vi "DDS_Clock.vi"() -> ()   [LabVIEW 2016] (continued)
CH0"=319000000.0, "CH1"=FALSE, "rel. amplitude CH1"=1.0, "phase [°] CH1"=0.0, "f0 [Hz] CH1"=310000000.0, "f1 [Hz] CH1"=310000000.0}, {"STEP"=0, "time[ms]"=0.05, "time tolerance[us]"=0.01, "CH0"=TRUE, "rel. amplitude CH0"=1.0, "phase [°] CH0"=0.0, "f0 [Hz] CH0"=319000000.0, "f1 [Hz] CH0"=319200000.0, "CH1"=FALSE, "rel. amplitude CH1"=1.0, "phase [°] CH1"=0.0, "f0 [Hz] CH1"=310000000.0, "f1 [Hz] CH1"=310000000.0}, {"STEP"=0, "time[ms]"=0.05, "time tolerance[us]"=0.01, "CH0"=TRUE, "rel. amplitude CH0"=1.0, "phase [°] CH0"=0.0, "f0 [Hz] CH0"=319200000.0, "f1 [Hz] CH0"=319400000.0, "CH1"=FALSE, "rel. amplitude CH1"=1.0, "phase [°] CH1"=0.0, "f0 [Hz] CH1"=310000000.0, "f1 [Hz] CH1"=310000000.0}, {"STEP"=0, "time[ms]"=0.05, "time tolerance[us]"=0.01, "CH0"=TRUE, "rel. amplitude CH0"=1.0, "phase [°] CH0"=0.0, "f0 [Hz] CH0"=319400000.0, "f1 [Hz] CH0"=319600000.0, "CH1"=FALSE, "rel. amplitude CH1"=1.0, "phase [°] CH1"=0.0, "f0 [Hz] CH1"=310000000.0, "f1 [Hz] CH1"=310000000.0}, {"STEP"=0, "time[ms]"=0.05, "time tolerance[us]"=0.01, "CH0"=TRUE, "rel. amplitude CH0"=1.0, "phase [°] CH0"=0.0, "f0 [Hz] CH0"=319600000.0, "f1 [Hz] CH0"=319800000.0, "CH1"=FALSE, "rel. amplitude CH1"=1.0, "phase [°] CH1"=0.0, "f0 [Hz] CH1"=310000000.0, "f1 [Hz] CH1"=310000000.0}, {"STEP"=0, "time[ms]"=0.05, "time tolerance[us]"=0.01, "CH0"=TRUE, "rel. amplitude CH0"=1.0, "phase [°] CH0"=0.0, "f0 [Hz] CH0"=319800000.0, "f1 [Hz] CH0"=320000000.0, "CH1"=FALSE, "rel. amplitude CH1"=1.0, "phase [°] CH1"=0.0, "f0 [Hz] CH1"=310000000.0, "f1 [Hz] CH1"=310000000.0}, {"STEP"=0, "time[ms]"=0.05, "time tolerance[us]"=0.01, "CH0"=TRUE, "rel. amplitude CH0"=1.0, "phase [°] CH0"=0.0, "f0 [Hz] CH0"=320000000.0, "f1 [Hz] CH0"=319800000.0, "CH1"=FALSE, "rel. amplitude CH1"=1.0, "phase [°] CH1"=0.0, "f0 [Hz] CH1"=310000000.0, "f1 [Hz] CH1"=310000000.0}, {"STEP"=0, "time[ms]"=0.05, "time tolerance[us]"=0.01, "CH0"=TRUE, "rel. amplitude CH0"=1.0, "phase [°] CH0"=0.0, "f0 [Hz] CH0"=319800000.0, "f1 [Hz] CH0"=319600000.0, "CH1"=FALSE, "rel. amplitude CH1"=1.0, "phase [°] CH1"=0.0, "f0 [Hz] CH1"=310000000.0, "f1 [Hz] CH1"=310000000.0}, {"STEP"=0, "time[ms]"=0.05, "time tolerance[us]"=0.01, "CH0"=TRUE, "rel. amplitude CH0"=1.0, "phase [°] CH0"=0.0, "f0 [Hz] CH0"=319600000.0, "f1 [Hz] CH0"=319400000.0, "CH1"=FALSE, "rel. amplitude CH1"=1.0, "phase [°] CH1"=0.0, "f0 [Hz] CH1"=310000000.0, "f1 [Hz] CH1"=310000000.0}, {"STEP"=0, "time[ms]"=0.05, "time tolerance[us]"=0.01, "CH0"=TRUE, "rel. amplitude CH0"=1.0, "phase [°] CH0"=0.0, "f0 [Hz] CH0"=319400000.0, "f1 [Hz] CH0"=319200000.0, "CH1"=FALSE, "rel. amplitude CH1"=1.0, "phase [°] CH1"=0.0, "f0 [Hz] CH1"=310000000.0, "f1 [Hz] CH1"=310000000.0}, {"STEP"=0, "time[ms]"=0.05, "time tolerance[us]"=0.01, "CH0"=TRUE, "rel. amplitude CH0"=1.0, "phase [°] CH0"=0.0, "f0 [Hz] CH0"=319200000.0, "f1 [Hz] CH0"=319000000.0, "CH1"=FALSE, "rel. amplitude CH1"=1.0, "phase [°] CH1"=0.0, "f0 [Hz] CH1"=310000000.0, "f1 [Hz] CH1"=310000000.0}, {"STEP"=0, "time[ms]"=0.05, "time tolerance[us]"=0.01, "CH0"=TRUE, "rel. amplitude CH0"=1.0, "phase [°] CH0"=0.0, "f0 [Hz] CH0"=319000000.0, "f1 [Hz] CH0"=318800000.0, "CH1"=FALSE, "rel. amplitude CH1"=1.0, "phase [°] CH1"=0.0, "f0 [Hz] CH1"=310000000.0, "f1 [Hz] CH1"=310000000.0}, {"STEP"=0, "time[ms]"=0.05, "time tolerance[us]"=0.01, "CH0"=TRUE, "rel. amplitude CH0"=1.0, "phase [°] CH0"=0.0, "f0 [Hz] CH0"=318800000.0, "f1 [Hz] CH0"=318600000.0, "CH1"=FALSE, "rel. amplitude CH1"=1.0, "phase [°] CH1"=0.0, "f0 [Hz] CH1"=310000000.0, "f1 [Hz] CH1"=310000000.0}, {"STEP"=0, "time[ms]"=0.05, "time tolerance[us]"=0.01, "CH0"=TRUE, "rel. amplitude CH0"=1.0, "phase [°] CH0"=0.0, "f0 [Hz] CH0"=318600000.0, "f1 [Hz] CH0"=318400000.0, "CH1"=FALSE, "rel. amplitude CH1"=1.0, "phase [°] CH1"=0.0, "f0 [Hz] CH1"=310000000.0, "f1 [Hz] CH1"=310000000.0}, {"STEP"=0, "time[ms]"=0.05, "time tolerance[us]"=0.01, "CH0"=TRUE, "rel. amplitude CH0"=1.0, "phase [°] CH0"=0.0, "f0 [Hz] CH0"=318400000.0, "f1 [Hz] CH0"=318200000.0, "CH1"=FALSE, "rel. amplitude CH1"=1.0, "phase [°] CH1"=0.0, "f0 [Hz] CH1"=310000000.0, "f1 [Hz] CH1"=310000000.0}, {"STEP"=0, "time[ms]"=0.05, "time tolerance[us]"=0.01, "CH0"=TRUE, "rel. amplitude CH0"=1.0, "phase [°] CH0"=0.0, "f0 [Hz] CH0"=318200000.0, "f1 [Hz] CH0"=318000000.0, "CH1"=FALSE, "rel. amplitude CH1"=1.0, "phase [°] CH1"=0.0, "f0 [Hz] CH1"=310000000.0, "f1 [Hz] CH1"=310000000.0}, {"STEP"=0, "time[ms]"=0.05, "time tolerance[us]"=0.01, "CH0"=TRUE, "rel. amplitude CH0"=1.0, "phase [°] CH0"=0.0, "f0 [Hz] CH0"=318000000.0, "f1 [Hz] CH0"=317800000.0, "CH1"=FALSE, "rel. amplitude CH1"=1.0, "phase [°] CH1"=0.0, "f0 [Hz] CH1"=310000000.0, "f1 [Hz] CH1"=310000000.0}, {"STEP"=0, "time[ms]"=0.05, "time tolerance[us]"=0.01, "CH0"=TRUE, "rel. amplitude CH0"=1.0, "phase [°] CH0"=0.0, "f0 [Hz] CH0"=317800000.0, "f1 [Hz] CH0"=317600000.0, "CH1"=FALSE, "rel. amplitude CH1"=1.0, "phase [°] CH1"=0.0, "f0 [Hz] CH1"=310000000.0, "f1 [Hz] CH1"=310000000.0}, {"STEP"=0, "time[ms]"=0.05, "time tolerance[us]"=0.01, "CH0"=TRUE, "rel. amplitude CH0"=1.0, "phase [°] CH0"=0.0, "f0 [Hz] CH0"=317600000.0, "f1 [Hz] CH0"=317400000.0, "CH1"=FALSE, "rel. amplitude CH1"=1.0, "phase [°] CH1"=0.0, "f0 [Hz] CH1"=310000000.0, "f1 [Hz] CH1"=310000000.0}, {"STEP"=0, "time[ms]"=0.05, "time tolerance[us]"=0.01, "CH0"=TRUE, "rel. amplitude CH0"=1.0, "phase [°] CH0"=0.0, "f0 [Hz] CH0"=317400000.0, "f1 [Hz] CH0"=317200000.0, "CH1"=FALSE, "rel. amplitude CH1"=1.0, "phase [°] CH1"=0.0, "f0 [Hz] CH1"=310000000.0, "f1 [Hz] CH1"=310000000.0}, {"STEP"=0, "time[ms]"=0.05, "time tolerance[us]"=0.01, "CH0"=TRUE, "rel. amplitude CH0"=1.0, "phase [°] CH0"=0.0, "f0 [Hz] CH0"=317200000.0, "f1 [Hz] CH0"=317000000.0, "CH1"=FALSE, "rel. amplitude CH1"=1.0, "phase [°] CH1"=0.0, "f0 [Hz] CH1"=310000000.0, "f1 [Hz] CH1"=310000000.0}, {"STEP"=0, "time[ms]"=0.05, "time tolerance[us]"=0.01, "CH0"=TRUE, "rel. amplitude CH0"=1.0, "phase [°] CH0"=0.0, "f0 [Hz] CH0"=317000000.0, "f1 [Hz] CH0"=316800000.0, "CH1"=FALSE, "rel. amplitude CH1"=1.0, "phase [°] CH1"=0.0, "f0 [Hz] CH1"=310000000.0, "f1 [Hz] CH1"=310000000.0}, {"STEP"=0, "time[ms]"=0.05, "time tolerance[us]"=0.01, "CH0"=TRUE, "rel. amplitude CH0"=1.0, "phase [°] CH0"=0.0, "f0 [Hz] CH0"=316800000.0, "f1 [Hz] CH0"=316600000.0, "CH1"=FALSE, "rel. amplitude CH1"=1.0, "phase [°] CH1"=0.0, "f0 [Hz] CH1"=310000000.0, "f1 [Hz] CH1"=310000000.0}, {"STEP"=0, "time[ms]"=0.05, "time tolerance[us]"=0.01, "CH0"=TRUE, "rel. amplitude CH0"=1.0, "phase [°] CH0"=0.0, "f0 [Hz] CH0"=316600000.0, "f1 [Hz] CH0"=316400000.0, "CH1"=FALSE, "rel. amplitude CH1"=1.0, "phase [°] CH1"=0.0, "f0 [Hz] CH1"=310000000.0, "f1 [Hz] CH1"=310000000.0}, {"STEP"=0, "time[ms]"=0.05, "time tolerance[us]"=0.01, "CH0"=TRUE, "rel. amplitude CH0"=1.0, "phase [°] CH0"=0.0, "f0 [Hz] CH0"=316400000.0, "f1 [Hz] CH0"=316200000.0, "CH1"=FALSE, "rel. amplitude CH1"=1.0, "phase [°] CH1"=0.0, "f0 [Hz] CH1"=310000000.0, "f1 [Hz] CH1"=310000000.0}, {"STEP"=0, "time[ms]"=0.05, "time tolerance[us]"=0.01, "CH0"=TRUE, "rel. amplitude CH0"=1.0, "phase [°] CH0"=0.0, "f0 [Hz] CH0"=316200000.0, "f1 [Hz] CH0"=316000000.0, "CH1"=FALSE, "rel. amplitude CH1"=1.0, "phase [°] CH1"=0.0, "f0 [Hz] CH1"=310000000.0, "f1 [Hz] CH1"=310000000.0}, {"STEP"=0, "time[ms]"=0.05, "time tolerance[us]"=0.01, "CH0"=TRUE, "rel. amplitude CH0"=1.0, "phase [°] CH0"=0.0, "f0 [Hz] CH0"=316000000.0, "f1 [Hz] CH0"=315800000.0, "CH1"=FALSE, "rel. amplitude CH1"=1.0, "phase [°] CH1"=0.0, "f0 [Hz] CH1"=310000000.0, "f1 [Hz] CH1"=310000000.0}, {"STEP"=0, "time[ms]"=0.05, "time tolerance[us]"=0.01, "CH0"=TRUE, "rel. amplitude CH0"=1.0, "phase [°] CH0"=0.0, "f0 [Hz] CH0"=315800000.0, "f1 [Hz] CH0"=315600000.0, "CH1"=FALSE, "rel. amplitude CH1"=1.0, "phase [°] CH1"=0.0, "f0 [Hz] CH1"=310000000.0, "f1 [Hz] CH1"=310000000.0}, {"STEP"=0, "time[ms]"=0.05, "time tolerance[us]"=0.01, "CH0"=TRUE, "rel. amplitude CH0"=1.0, "phase [°] CH0"=0.0, "f0 [Hz] CH0"=315600000.0, "f1 [Hz] CH0"=315400000.0, "CH1"=FALSE, "rel. amplitude CH1"=1.0, "phase [°] CH1"=0.0, "f0 [Hz] CH1"=310000000.0, "f1 [Hz] CH1"=310000000.0}, {"STEP"=0, "time[ms]"=0.05, "time tolerance[us]"=0.01, "CH0"=TRUE, "rel. amplitude CH0"=1.0, "phase [°] CH0"=0.0, "f0 [Hz] CH0"=315400000.0, "f1 [Hz] CH0"=315200000.0, "CH1"=FALSE, "rel. amplitude CH1"=1.0, "phase [°] CH1"=0.0, "f0 [Hz] CH1"=310000000.0, "f1 [Hz] CH1"=310000000.0}, {"STEP"=0, "time[ms]"=0.05, "time tolerance[us]"=0.01, "CH0"=TRUE, "rel. amplitude CH0"=1.0, "phase [°] CH0"=0.0, "f0 [Hz] CH0"=315200000.0, "f1 [Hz] CH0"=315000000.0, "CH1"=FALSE, "rel. amplitude CH1"=1.0, "phase [°] CH1"=0.0, "f0 [Hz] CH1"=310000000.0, "f1 [Hz] CH1"=310000000.0}, {"STEP"=0, "time[ms]"=0.05, "time tolerance[us]"=0.01, "CH0"=TRUE, "rel. amplitude CH0"=1.0, "phase [°] CH0"=0.0, "f0 [Hz] CH0"=315000000.0, "f1 [Hz] CH0"=314800000.0, "CH1"=FALSE, "rel. amplitude CH1"=1.0, "phase [°] CH1"=0.0, "f0 [Hz] CH1"=310000000.0, "f1 [Hz] CH1"=310000000.0}, {"STEP"=0, "time[ms]"=0.05, "time tolerance[us]"=0.01, "CH0"=TRUE, "rel. amplitude CH0"=1.0, "phase [°] CH0"=0.0, "f0 [Hz] CH0"=314800000.0, "f1 [Hz] CH0"=314600000.0, "CH1"=FALSE, "rel. amplitude CH1"=1.0, "phase [°] CH1"=0.0, "f0 [Hz] CH1"=310000000.0, "f1 [Hz] CH1"=310000000.0}, {"STEP"=0, "time[ms]"=0.05, "time tolerance[us]"=0.01, "CH0"=TRUE, "rel. amplitude CH0"=1.0, "phase [°] CH0"=0.0, "f0 [Hz] CH0"=314600000.0, "f1 [Hz] CH0"=314400000.0, "CH1"=FALSE, "rel. amplitude CH1"=1.0, "phase [°] CH1"=0.0, "f0 [Hz] CH1"=310000000.0, "f1 [Hz] CH1"=310000000.0}, {"STEP"=0, "time[ms]"=0.05, "time tolerance[us]"=0.01, "CH0"=TRUE, "rel. amplitude CH0"=1.0, "phase [°] CH0"=0.0, "f0 [Hz] CH0"=314400000.0, "f1 [Hz] CH0"=314200000.0, "CH1"=FALSE, "rel. amplitude CH1"=1.0, "phase [°] CH1"=0.0, "f0 [Hz] CH1"=310000000.0, "f1 [Hz] CH1"=310000000.0}, {"STEP"=0, "time[ms]"=0.05, "time tolerance[us]"=0.01, "CH0"=TRUE, "rel. amplitude CH0"=1.0, "phase [°] CH0"=0.0, "f0 [Hz] CH0"=314200000.0, "f1 [Hz] CH0"=314000000.0, "CH1"=FALSE, "rel. amplitude CH1"=1.0, "phase [°] CH1"=0.0, "f0 [Hz] CH1"=310000000.0, "f1 [Hz] CH1"=310000000.0}, {"STEP"=0, "time[ms]"=0.05, "time tolerance[us]"=0.01, "CH0"=TRUE, "rel. amplitude CH0"=1.0, "phase [°] CH0"=0.0, "f0 [Hz] CH0"=314000000.0, "f1 [Hz] CH0"=313800000.0, "CH1"=FALSE, "rel. amplitude CH1"=1.0, "phase [°] CH1"=0.0, "f0 [Hz] CH1"=310000000.0, "f1 [Hz] CH1"=310000000.0}, {"STEP"=0, "time[ms]"=0.05, "time tolerance[us]"=0.01, "CH0"=TRUE, "rel. amplitude CH0"=1.0, "phase [°] CH0"=0.0, "f0 [Hz] CH0"=313800000.0, "f1 [Hz] CH0"=313600000.0, "CH1"=FALSE, "rel. amplitude CH1"=1.0, "phase [°] CH1"=0.0, "f0 [Hz] CH1"=310000000.0, "f1 [Hz] CH1"=310000000.0}, {"STEP"=0, "time[ms]"=0.05, "time tolerance[us]"=0.01, "CH0"=TRUE, "rel. amplitude CH0"=1.0, "phase [°] CH0"=0.0, "f0 [Hz] CH0"=313600000.0, "f1 [Hz] CH0"=313400000.0, "CH1"=FALSE, "rel. amplitude CH1"=1.0, "phase [°] CH1"=0.0, "f0 [Hz] CH1"=310000000.0, "f1 [Hz] CH1"=310000000.0}, {"STEP"=0, "time[ms]"=0.05, "time tolerance[us]"=0.01, "CH0"=TRUE, "rel. amplitude CH0"=1.0, "phase [°] CH0"=0.0, "f0 [Hz] CH0"=313400000.0, "f1 [Hz] CH0"=313200000.0, "CH1"=FALSE, "rel. amplitude CH1"=1.0, "phase [°] CH1"=0.0, "f0 [Hz] CH1"=310000000.0, "f1 [Hz] CH1"=310000000.0}, {"STEP"=0, "time[ms]"=0.05, "time tolerance[us]"=0.01, "CH0"=TRUE, "rel. amplitude CH0"=1.0, "phase [°] CH0"=0.0, "f0 [Hz] CH0"=313200000.0, "f1 [Hz] CH0"=313000000.0, "CH1"=FALSE, "rel. amplitude CH1"=1.0, "phase [°] CH1"=0.0, "f0 [Hz] CH1"=310000000.0, "f1 [Hz] CH1"=310000000.0}, {"STEP"=0, "time[ms]"=0.05, "time tolerance[us]"=0.01, "CH0"=TRUE, "rel. amplitude CH0"=1.0, "phase [°] CH0"=0.0, "f0 [Hz] CH0"=313000000.0, "f1 [Hz] CH0"=312800000.0, "CH1"=FALSE, "rel. amplitude CH1"=1.0, "phase [°] CH1"=0.0, "f0 [Hz] CH1"=310000000.0, "f1 [Hz] CH1"=310000000.0}, {"STEP"=0, "time[ms]"=0.05, "time tolerance[us]"=0.01, "CH0"=TRUE, "rel. amplitude CH0"=1.0, "phase [°] CH0"=0.0, "f0 [Hz] CH0"=312800000.0, "f1 [Hz] CH0"=312600000.0, "CH1"=FALSE, "rel. amplitude CH1"=1.0, "phase [°] CH1"=0.0, "f0 [Hz] CH1"=310000000.0, "f1 [Hz] CH1"=310000000.0}, {"STEP"=0, "time[ms]"=0.05, "time tolerance[us]"=0.01, "CH0"=TRUE, "rel. amplitude CH0"=1.0, "phase [°] CH0"=0.0, "f0 [Hz] CH0"=312600000.0, "f1 [Hz] CH0"=312400000.0, "CH1"=FALSE, "rel. amplitude CH1"=1.0, "phase [°] CH1"=0.0, "f0 [Hz] CH1"=310000000.0, "f1 [Hz] CH1"=310000000.0}, {"STEP"=0, "time[ms]"=0.05, "time tolerance[us]"=0.01, "CH0"=TRUE, "rel. amplitude CH0"=1.0, "phase [°] CH0"=0.0, "f0 [Hz] CH0"=312400000.0, "f1 [Hz] CH0"=312200000.0, "CH1"=FALSE, "rel. amplitude CH1"=1.0, "phase [°] CH1"=0.0, "f0 [Hz] CH1"=310000000.0, "f1 [Hz] CH1"=310000000.0}, {"STEP"=0, "time[ms]"=0.05, "time tolerance[us]"=0.01, "CH0"=TRUE, "rel. amplitude CH0"=1.0, "phase [°] CH0"=0.0, "f0 [Hz] CH0"=312200000.0, "f1 [Hz] CH0"=312000000.0, "CH1"=FALSE, "rel. amplitude CH1"=1.0, "phase [°] CH1"=0.0, "f0 [Hz] CH1"=310000000.0, "f1 [Hz] CH1"=310000000.0}, {"STEP"=0, "time[ms]"=0.05, "time tolerance[us]"=0.01, "CH0"=TRUE, "rel. amplitude CH0"=1.0, "phase [°] CH0"=0.0, "f0 [Hz] CH0"=312000000.0, "f1 [Hz] CH0"=311800000.0, "CH1"=FALSE, "rel. amplitude CH1"=1.0, "phase [°] CH1"=0.0, "f0 [Hz] CH1"=310000000.0, "f1 [Hz] CH1"=310000000.0}, {"STEP"=0, "time[ms]"=0.05, "time tolerance[us]"=0.01, "CH0"=TRUE, "rel. amplitude CH0"=1.0, "phase [°] CH0"=0.0, "f0 [Hz] CH0"=311800000.0, "f1 [Hz] CH0"=311600000.0, "CH1"=FALSE, "rel. amplitude CH1"=1.0, "phase [°] CH1"=0.0, "f0 [Hz] CH1"=310000000.0, "f1 [Hz] CH1"=310000000.0}, {"STEP"=0, "time[ms]"=0.05, "time tolerance[us]"=0.01, "CH0"=TRUE, "rel. amplitude CH0"=1.0, "phase [°] CH0"=0.0, "f0 [Hz] CH0"=311600000.0, "f1 [Hz] CH0"=311400000.0, "CH1"=FALSE, "rel. amplitude CH1"=1.0, "phase [°] CH1"=0.0, "f0 [Hz] CH1"=310000000.0, "f1 [Hz] CH1"=310000000.0}, {"STEP"=0, "time[ms]"=0.05, "time tolerance[us]"=0.01, "CH0"=TRUE, "rel. amplitude CH0"=1.0, "phase [°] CH0"=0.0, "f0 [Hz] CH0"=311400000.0, "f1 [Hz] CH0"=311200000.0, "CH1"=FALSE, "rel. amplitude CH1"=1.0, "phase [°] CH1"=0.0, "f0 [Hz] CH1"=310000000.0, "f1 [Hz] CH1"=310000000.0}, {"STEP"=0, "time[ms]"=0.05, "time tolerance[us]"=0.01, "CH0"=TRUE, "rel. amplitude CH0"=1.0, "phase [°] CH0"=0.0, "f0 [Hz] CH0"=311200000.0, "f1 [Hz] CH0"=311000000.0, "CH1"=FALSE, "rel. amplitude CH1"=1.0, "phase [°] CH1"=0.0, "f0 [Hz] CH1"=310000000.0, "f1 [Hz] CH1"=310000000.0}, {"STEP"=0, "time[ms]"=0.05, "time tolerance[us]"=0.01, "CH0"=TRUE, "rel. amplitude CH0"=1.0, "phase [°] CH0"=0.0, "f0 [Hz] CH0"=311000000.0, "f1 [Hz] CH0"=310800000.0, "CH1"=FALSE, "rel. amplitude CH1"=1.0, "phase [°] CH1"=0.0, "f0 [Hz] CH1"=310000000.0, "f1 [Hz] CH1"=310000000.0}, {"STEP"=0, "time[ms]"=0.05, "time tolerance[us]"=0.01, "CH0"=TRUE, "rel. amplitude CH0"=1.0, "phase [°] CH0"=0.0, "f0 [Hz] CH0"=310800000.0, "f1 [Hz] CH0"=310600000.0, "CH1"=FALSE, "rel. amplitude CH1"=1.0, "phase [°] CH1"=0.0, "f0 [Hz] CH1"=310000000.0, "f1 [Hz] CH1"=310000000.0}, {"STEP"=0, "time[ms]"=0.05, "time tolerance[us]"=0.01, "CH0"=TRUE, "rel. amplitude CH0"=1.0, "phase [°] CH0"=0.0, "f0 [Hz] CH0"=310600000.0, "f1 [Hz] CH0"=310400000.0, "CH1"=FALSE, "rel. amplitude CH1"=1.0, "phase [°] CH1"=0.0, "f0 [Hz] CH1"=310000000.0, "f1 [Hz] CH1"=310000000.0}, {"STEP"=0, "time[ms]"=0.05, "time tolerance[us]"=0.01, "CH0"=TRUE, "rel. amplitude CH0"=1.0, "phase [°] CH0"=0.0, "f0 [Hz] CH0"=310400000.0, "f1 [Hz] CH0"=310200000.0, "CH1"=FALSE, "rel. amplitude CH1"=1.0, "phase [°] CH1"=0.0, "f0 [Hz] CH1"=310000000.0, "f1 [Hz] CH1"=310000000.0}, {"STEP"=0, "time[ms]"=0.05, "time tolerance[us]"=0.01, "CH0"=TRUE, "rel. amplitude CH0"=1.0, "phase [°] CH0"=0.0, "f0 [Hz] CH0"=310200000.0, "f1 [Hz] CH0"=310000000.0, "CH1"=FALSE, "rel. amplitude CH1"=1.0, "phase [°] CH1"=0.0, "f0 [Hz] CH1"=310000000.0, "f1 [Hz] CH1"=310000000.0}, {"STEP"=0, "time[ms]"=0.05, "time tolerance[us]"=0.01, "CH0"=TRUE, "rel. amplitude CH0"=1.0, "phase [°] CH0"=0.0, "f0 [Hz] CH0"=310000000.0, "f1 [Hz] CH0"=309800000.0, "CH1"=FALSE, "rel. amplitude CH1"=1.0, "phase [°] CH1"=0.0, "f0 [Hz] CH1"=310000000.0, "f1 [Hz] CH1"=310000000.0}, {"STEP"=0, "time[ms]"=0.05, "time tolerance[us]"=0.01, "CH0"=TRUE, "rel. amplitude CH0"=1.0, "phase [°] CH0"=0.0, "f0 [Hz] CH0"=309800000.0, "f1 [Hz] CH0"=309600000.0, "CH1"=FALSE, "rel. amplitude CH1"=1.0, "phase [°] CH1"=0.0, "f0 [Hz] CH1"=310000000.0, "f1 [Hz] CH1"=310000000.0}, {"STEP"=0, "time[ms]"=0.05, "time tolerance[us]"=0.01, "CH0"=TRUE, "rel. amplitude CH0"=1.0, "phase [°] CH0"=0.0, "f0 [Hz] CH0"=309600000.0, "f1 [Hz] CH0"=309400000.0, "CH1"=FALSE, "rel. amplitude CH1"=1.0, "phase [°] CH1"=0.0, "f0 [Hz] CH1"=310000000.0, "f1 [Hz] CH1"=310000000.0}, {"STEP"=0, "time[ms]"=0.05, "time tolerance[us]"=0.01, "CH0"=TRUE, "rel. amplitude CH0"=1.0, "phase [°] CH0"=0.0, "f0 [Hz] CH0"=309400000.0, "f1 [Hz] CH0"=309200000.0, "CH1"=FALSE, "rel. amplitude CH1"=1.0, "phase [°] CH1"=0.0, "f0 [Hz] CH1"=310000000.0, "f1 [Hz] CH1"=310000000.0}, {"STEP"=0, "time[ms]"=0.05, "time tolerance[us]"=0.01, "CH0"=TRUE, "rel. amplitude CH0"=1.0, "phase [°] CH0"=0.0, "f0 [Hz] CH0"=309200000.0, "f1 [Hz] CH0"=309000000.0, "CH1"=FALSE, "rel. amplitude CH1"=1.0, "phase [°] CH1"=0.0, "f0 [Hz] CH1"=310000000.0, "f1 [Hz] CH1"=310000000.0}, {"STEP"=0, "time[ms]"=0.05, "time tolerance[us]"=0.01, "CH0"=TRUE, "rel. amplitude CH0"=1.0, "phase [°] CH0"=0.0, "f0 [Hz] CH0"=309000000.0, "f1 [Hz] CH0"=308800000.0, "CH1"=FALSE, "rel. amplitude CH1"=1.0, "phase [°] CH1"=0.0, "f0 [Hz] CH1"=310000000.0, "f1 [Hz] CH1"=310000000.0}, {"STEP"=0, "time[ms]"=0.05, "time tolerance[us]"=0.01, "CH0"=TRUE, "rel. amplitude CH0"=1.0, "phase [°] CH0"=0.0, "f0 [Hz] CH0"=308800000.0, "f1 [Hz] CH0"=308600000.0, "CH1"=FALSE, "rel. amplitude CH1"=1.0, "phase [°] CH1"=0.0, "f0 [Hz] CH1"=310000000.0, "f1 [Hz] CH1"=310000000.0}, {"STEP"=0, "time[ms]"=0.05, "time tolerance[us]"=0.01, "CH0"=TRUE, "rel. amplitude CH0"=1.0, "phase [°] CH0"=0.0, "f0 [Hz] CH0"=308600000.0, "f1 [Hz] CH0"=308400000.0, "CH1"=FALSE, "rel. amplitude CH1"=1.0, "phase [°] CH1"=0.0, "f0 [Hz] CH1"=310000000.0, "f1 [Hz] CH1"=310000000.0}, {"STEP"=0, "time[ms]"=0.05, "time tolerance[us]"=0.01, "CH0"=TRUE, "rel. amplitude CH0"=1.0, "phase [°] CH0"=0.0, "f0 [Hz] CH0"=308400000.0, "f1 [Hz] CH0"=308200000.0, "CH1"=FALSE, "rel. amplitude CH1"=1.0, "phase [°] CH1"=0.0, "f0 [Hz] CH1"=310000000.0, "f1 [Hz] CH1"=310000000.0}, {"STEP"=0, "time[ms]"=0.05, "time tolerance[us]"=0.01, "CH0"=TRUE, "rel. amplitude CH0"=1.0, "phase [°] CH0"=0.0, "f0 [Hz] CH0"=308200000.0, "f1 [Hz] CH0"=308000000.0, "CH1"=FALSE, "rel. amplitude CH1"=1.0, "phase [°] CH1"=0.0, "f0 [Hz] CH1"=310000000.0, "f1 [Hz] CH1"=310000000.0}, {"STEP"=0, "time[ms]"=0.05, "time tolerance[us]"=0.01, "CH0"=TRUE, "rel. amplitude CH0"=1.0, "phase [°] CH0"=0.0, "f0 [Hz] CH0"=308000000.0, "f1 [Hz] CH0"=307800000.0, "CH1"=FALSE, "rel. amplitude CH1"=1.0, "phase [°] CH1"=0.0, "f0 [Hz] CH1"=310000000.0, "f1 [Hz] CH1"=310000000.0}, {"STEP"=0, "time[ms]"=0.05, "time tolerance[us]"=0.01, "CH0"=TRUE, "rel. amplitude CH0"=1.0, "phase [°] CH0"=0.0, "f0 [Hz] CH0"=307800000.0, "f1 [Hz] CH0"=307600000.0, "CH1"=FALSE, "rel. amplitude CH1"=1.0, "phase [°] CH1"=0.0, "f0 [Hz] CH1"=310000000.0, "f1 [Hz] CH1"=310000000.0}, {"STEP"=0, "time[ms]"=0.05, "time tolerance[us]"=0.01, "CH0"=TRUE, "rel. amplitude CH0"=1.0, "phase [°] CH0"=0.0, "f0 [Hz] CH0"=307600000.0, "f1 [Hz] CH0"=307400000.0, "CH1"=FALSE, "rel. amplitude CH1"=1.0, "phase [°] CH1"=0.0, "f0 [Hz] CH1"=310000000.0, "f1 [Hz] CH1"=310000000.0}, {"STEP"=0, "time[ms]"=0.05, "time tolerance[us]"=0.01, "CH0"=TRUE, "rel. amplitude CH0"=1.0, "phase [°] CH0"=0.0, "f0 [Hz] CH0"=307400000.0, "f1 [Hz] CH0"=307200000.0, "CH1"=FALSE, "rel. amplitude CH1"=1.0, "phase [°] CH1"=0.0, "f0 [Hz] CH1"=310000000.0, "f1 [Hz] CH1"=310000000.0}, {"STEP"=0, "time[ms]"=0.05, "time tolerance[us]"=0.01, "CH0"=TRUE, "rel. amplitude CH0"=1.0, "phase [°] CH0"=0.0, "f0 [Hz] CH0"=307200000.0, "f1 [Hz] CH0"=307000000.0, "CH1"=FALSE, "rel. amplitude CH1"=1.0, "phase [°] CH1"=0.0, "f0 [Hz] CH1"=310000000.0, "f1 [Hz] CH1"=310000000.0}, {"STEP"=0, "time[ms]"=0.05, "time tolerance[us]"=0.01, 
